vi "Read Pic Width.vi"(8 "error in":errorcluster, 11 "Popup in":refnum<class "Popup.lvclass">) -> (0 "error out":errorcluster, 2 "Pic Width":i16, 3 "Popup out":refnum<class "Popup.lvclass">)   [LabVIEW 2021, in "Pop-Up.lvlib" / "Popup.lvclass"]
doc: "Read the width of the custom picture\n\n<b>Code Developed By:</b> +\nDaniel Coons +\nhttps://github.com/danielcoons/tsc-pop-up"
uses:
  Popup.lvclass
  Popup.lvclass/Popup.ctl
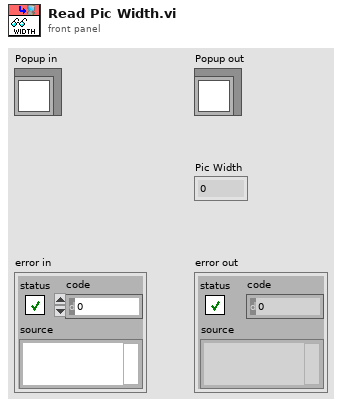
[diagram p1: front panel]
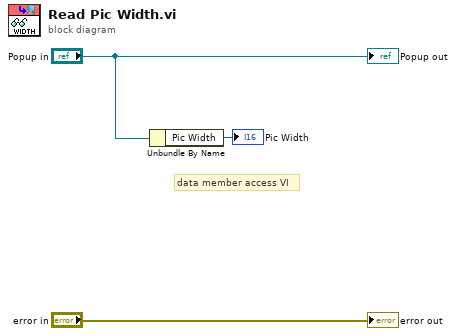
[diagram p0: block diagram]
diagram:
  # "data member access VI"
  n1 = Unbundle By Name("Popup in") -> ("Pic Width"=→"Pic Width":i16)
  "error out" <- "error in"
  "Popup out" <- "Popup in"
